vi "Ejercicio_18_ARDUINO_DAQ_SERVO.vi"() -> ()   [LabVIEW 2020]
uses:
  <vilib>/Instr/_visa.llb/VISA Configure Serial Port (Instr).vi
panel:
  in  "VISA resource name":refnum<visa-resource-name>
  out "concatenated string":string
  out "Waveform Graph":dynamicdata(graph)
  in  "Duty Cycle (%)":dbl=50.0
  in  "stop":bool
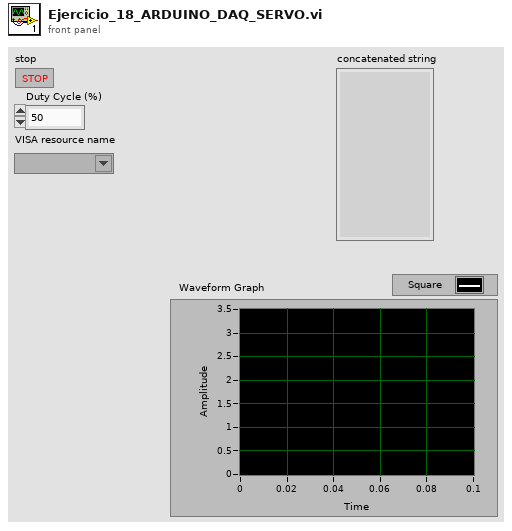
[diagram p1: front panel]
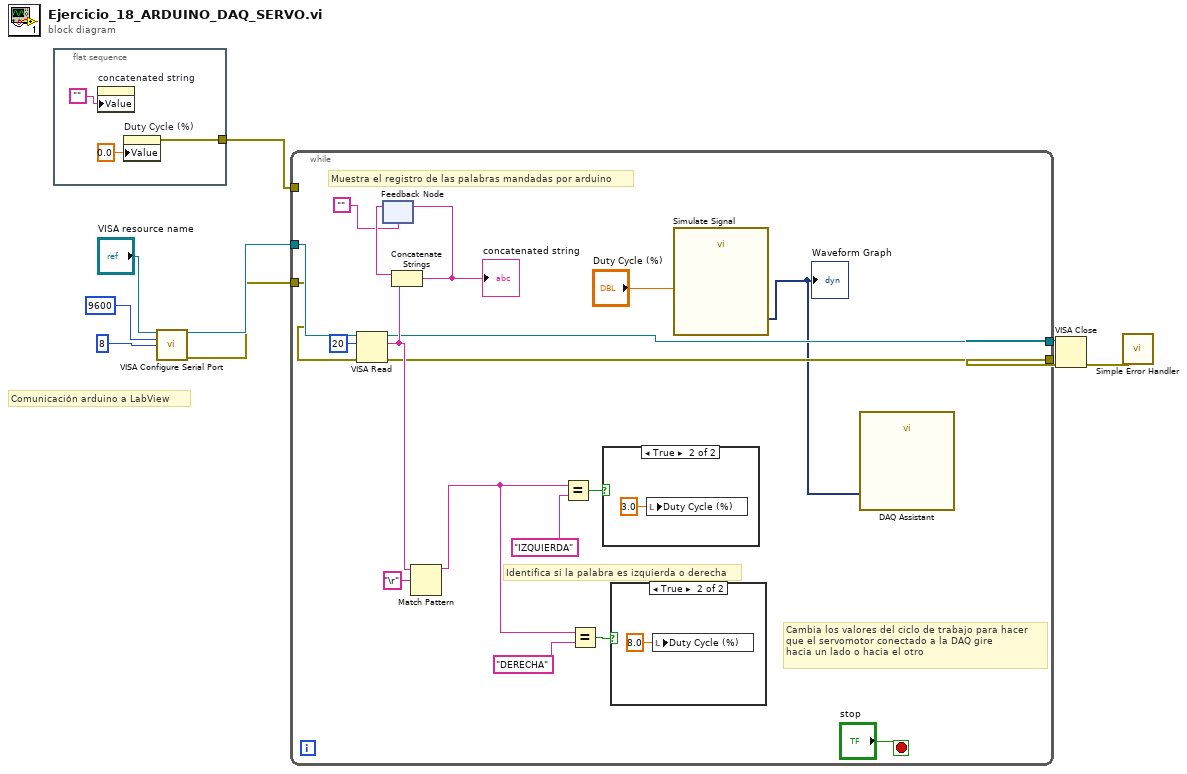
[diagram p0: block diagram]
diagram:
  # "Comunicación arduino a LabView"
  n1 = flat-sequence {
    tunnel: [w10] -> w4
    frame #0 {
      n2 = property on="concatenated string" class="Str"("Value"="") -> ()  [unwired: 2 in, 2 out]
      n3 = property on="Duty Cycle (%)" class="DigNum (strict)"("Value"=0.0 ("Duty Cycle (%)")) -> (error out=w10:errorcluster)  [unwired: 2 in, 1 out]
    }
  }
  n4 = call-poly "VISA Configure Serial Port"("VISA resource name"="VISA resource name", "baud rate (9600)"=u32 9600, "data bits (8)"=u16 8) -> ("VISA resource name out"=w9:refnum<visa-resource-name>, "error out"=w8:errorcluster)  [unwired: 11 in]
  n5 = while {
    tunnel: w9 -> [w19]
    tunnel: w8 -> [w18]
    tunnel: [w15] -> w3
    tunnel: w4 -> [_]
    tunnel: [w14] -> w2
    stop <- "stop" stop-if-true
    # "Cambia los valores del ciclo de trabajo para hacer\nque el servomotor conectado a la DAQ gire\nhacia un lado o hacia el otro"
    # "Identifica si la palabra es izquierda o derecha"
    # "Muestra el registro de las palabras mandadas por arduino"
    n6 = VISA Read(VISA resource name=w19, byte count=u32 20, error in (no error)=w18) -> (VISA resource name out=w14:refnum<visa-resource-name>, read buffer=w16:string, error out=w15:errorcluster)  [unwired: 1 out]
    n7 = feedback #1("") -> (w27:string)
    n8 = Concatenate Strings(w27, w16) -> (w28:string)
    "concatenated string" <- w28
    n9 = feedback-in #1(w28) -> ()
    n10 = Match Pattern(string=w16, regular expression="\r") -> (before substring=w23:string)  [unwired: 1 in, 3 out]
    n11 = Equal?(x=w23, y="IZQUIERDA") -> (x = y?=w25:bool)
    n12 = Equal?(x=w23, y="DERECHA") -> (x = y?=w24:bool)
    n13 = case shown="True" w25 {
      frame False {
      }
      frame True {
        n14 = local write "Duty Cycle (%)"(3.0 ("Duty Cycle (%)")) -> ()
      }
    }
    n15 = case shown="True" w24 {
      frame False {
      }
      frame True {
        n16 = local write "Duty Cycle (%)"(8.0 ("Duty Cycle (%)")) -> ()
      }
    }
    n17 = call "Simulate Signal"("Duty Cycle (%)"="Duty Cycle (%)") -> ("Square"=w13:dynamicdata)  [unwired: 13 in, 1 out]
    "Waveform Graph" <- w13
    n18 = call "DAQ Assistant"("data"=w13) -> ()  [unwired: 17 in, 2 out]
  }
  n19 = VISA Close(VISA resource name=w2, error in (no error)=w3) -> (error out=w1:errorcluster)
  n20 = call <vilib>:"Simple Error Handler.vi"("error in (no error)"=w1) -> ()  [unwired: 4 in, 5 out]
